vi "Modify Reaction To Error.vi"(6 "Priority (F)":bool, 8 "error in (no error)":errorcluster, 11 "Data":variant) -> (0 "error out":errorcluster)   [LabVIEW 2020, in "Error Handler.lvlib"]
uses:
  Error Handler.lvlib
  Private Controls/Element.ctl
  Private Controls/Module Action.ctl
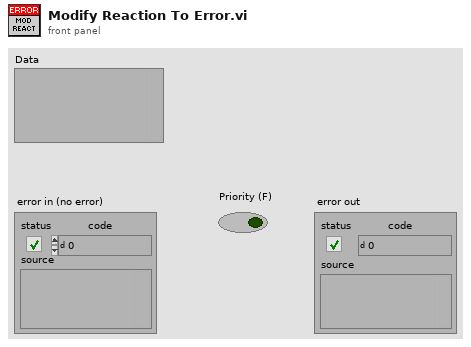
[diagram p1: front panel]
types:
  T1 = typedef "Error Handler.lvlib/Module Action.ctl" = enum16{"Initialise Module", "Modify Reaction to Error", "Log to File", "Prompt User", "External Error", "Internal Error", "Exit"}
  T2 = typedef "Error Handler.lvlib/Element.ctl" = cluster{"Action":T1, "Data":variant}
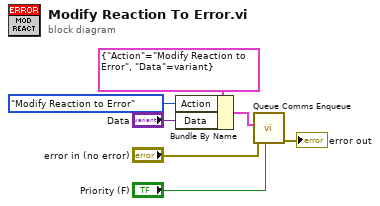
[diagram p0: block diagram]
diagram:
  n1 = Bundle By Name(cluster=T2 {"Action"=enum."Modify Reaction to Error", "Data"=variant} ("Element"), "Action"=Module_Action."Modify Reaction to Error", "Data"="Data") -> (w1:T2)
  n2 = call "Queue Comms Enqueue.vi"("Priority (F)"="Priority (F)", "error in (no error)"="error in (no error)", "Element"=w1) -> ("error out"=→"error out":errorcluster)  [unwired: 8 in]
